vi "בדיקת מתח תפיסה של סליל פיקוד ללא עומס 4.vi"(8 "error":errorcluster, 11 "Path for Log":path) -> (0 "error out":errorcluster, 1 "מצב ממסר פתוח/סגור":bool, 2 "מתח סגירת הממסר":dbl format="%.4f", 3 "מתח מוצא מהספק":dbl format="%.4f", 5 "resultUserPrompt":bool)   [LabVIEW 2014]
uses:
  <vilib>/DAQmx/create/channels.llb/DAQmx Create Channel (DO-Digital Output).vi
  <vilib>/DAQmx/write.llb/DAQmx Write (Digital Bool 1Line 1Point).vi
panel:
  out "progress":dbl(slide) scale=0.0..36.0
  out "error IO DMM":errorcluster
  in  "Stop Button":bool
  # "Right-Click to\nexplain error"
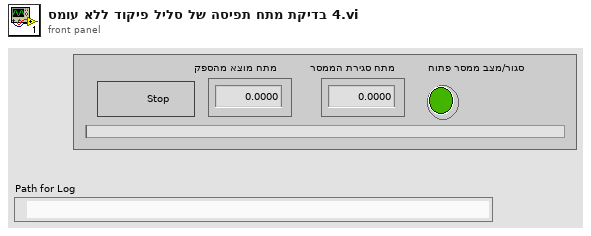
[diagram p1: front panel]
types:
  T1 = enum32{"Invalid", "Standard", "Closed", "Hidden", "Minimized", "Maximized"}
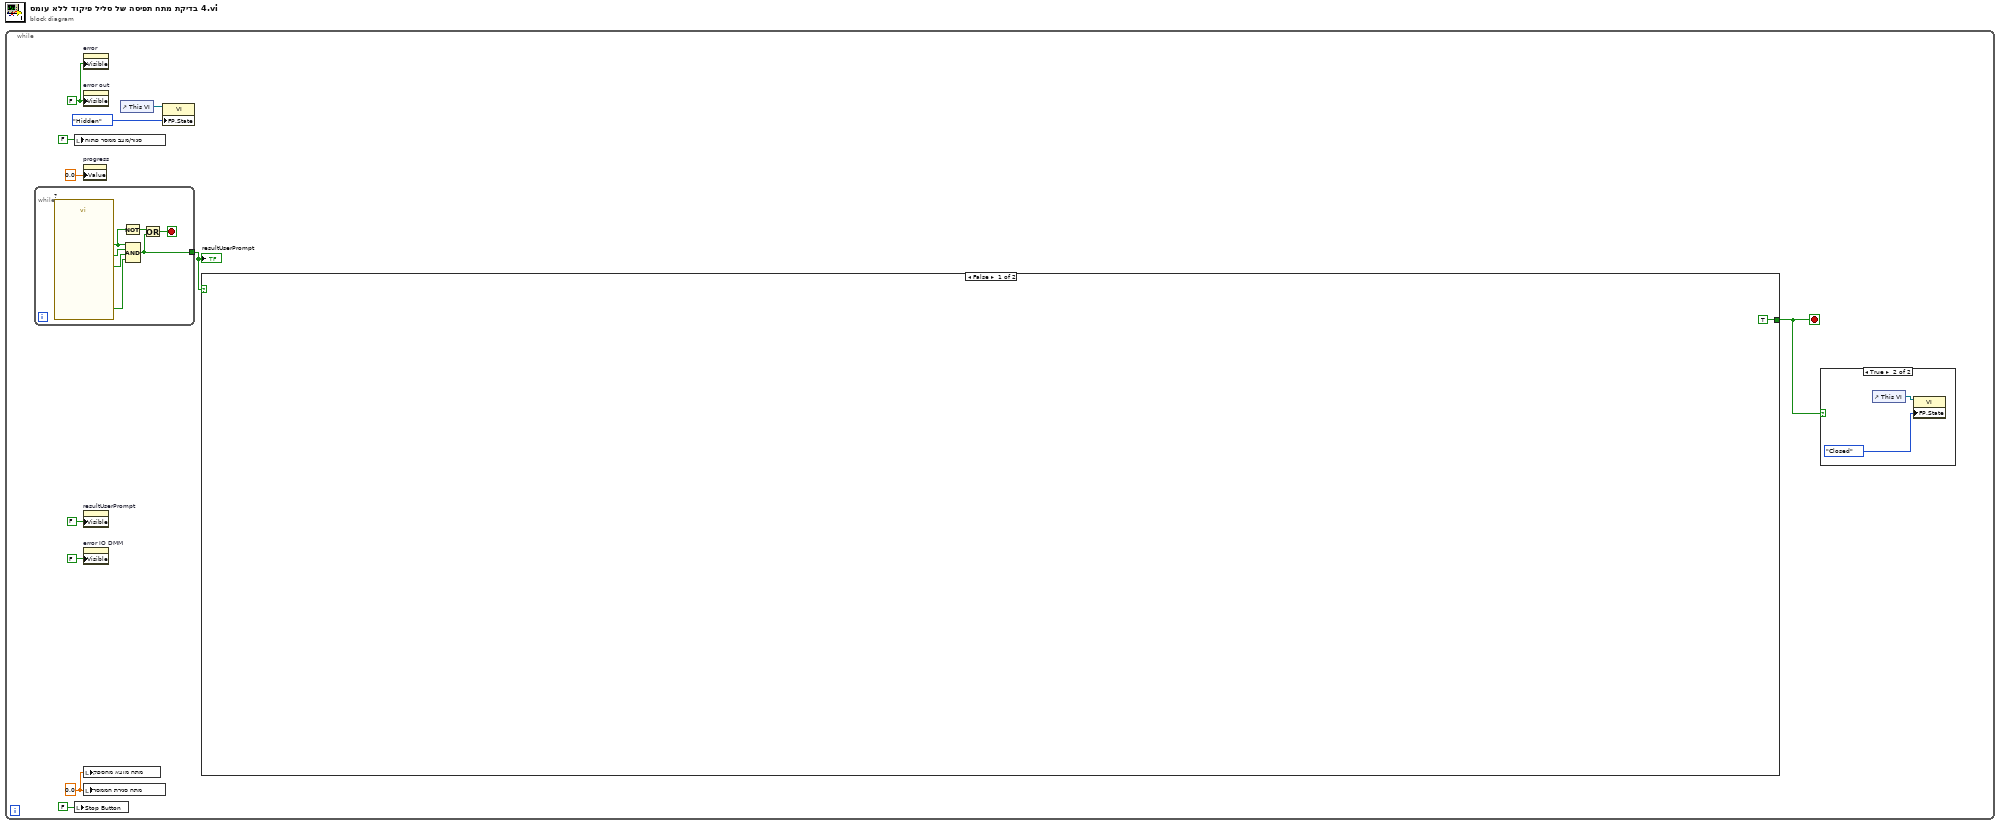
[diagram p0: block diagram]
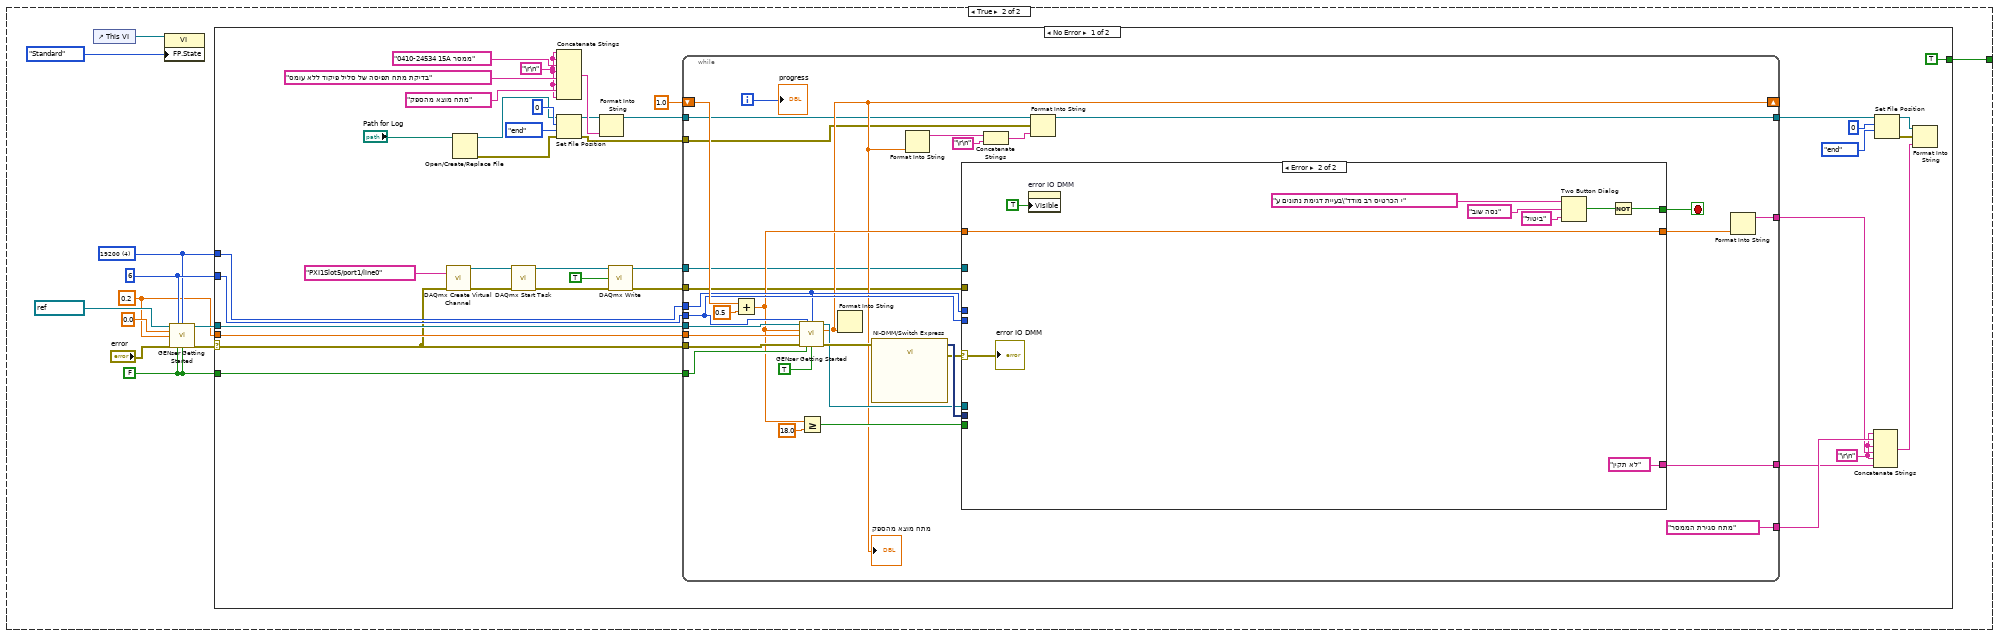
[diagram p3: hidden frame]
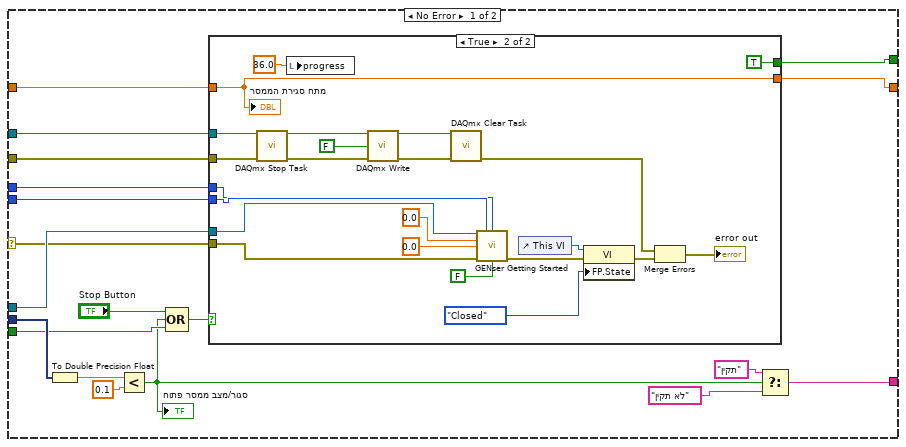
[diagram p4: hidden frame]
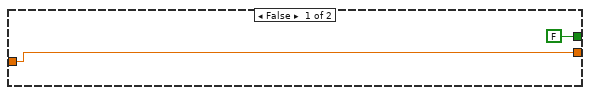
[diagram p5: hidden frame]
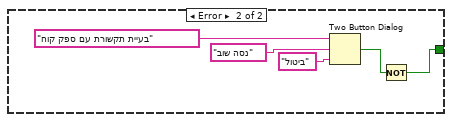
[diagram p6: hidden frame]
diagram:
  n1 = while {
    stop <- w1 stop-if-true
    w3 = FALSE ("Visible")
    w6 = 0.0 ("signals out")
    n2 = while {
      tunnel: [w12] -> w11
      stop <- w15 stop-if-true
      n3 = call "?"() -> ("הדקי הרב מודד"=w16:bool, "(מגע שלילי (מעטפת"=w17:bool, "A מגע חיובי"=w18:bool, "OK"=w13:bool)  [unwired: 15 in, 1 out]
      n4 = Not(x=w13) -> (.not. x?=w14:bool)
      n5 = Compound Arithmetic op=AND(w13, w18, w17, w16) -> (w12:bool)
      n6 = Or(x=w14, y=w12) -> (x .or. y?=w15:bool)
    }
    "resultUserPrompt" <- w11
    n7 = local write "מצב ממסר פתוח/סגור"(FALSE ("מגע סגור")) -> ()
    n8 = local write "Stop Button"(FALSE ("Reset (T)")) -> ()
    n9 = property on="error" class="Clust (strict)"("Visible"=w3) -> ()  [unwired: 2 in, 2 out]
    n10 = property on="error out" class="Clust (strict)"("Visible"=w3) -> ()  [unwired: 2 in, 2 out]
    n11 = property on="progress" class="Slide (strict)"("Value"=0.0 ("progress")) -> ()  [unwired: 2 in, 2 out]
    n12 = property on="resultUserPrompt" class="Bool (strict)"("Visible"=FALSE) -> ()  [unwired: 2 in, 2 out]
    n13 = property on="error IO DMM" class="Clust (strict)"("Visible"=FALSE) -> ()  [unwired: 2 in, 2 out]
    n14 = local write "מתח מוצא מהספק"(w6) -> ()
    n15 = local write "מתח סגירת הממסר"(w6) -> ()
    n16 = control-ref of="This VI"() -> (w5:refnum<vi>)
    n17 = property class="VI"(reference=w5, "FP.State"=T1."Hidden" ("Front Panel Window:State")) -> ()  [unwired: 1 in, 2 out]
    n18 = case shown="False" w11 {
      tunnel: [TRUE ("T button?") w27] -> w1
      frame False {
      }
      frame True {
        w26 = FALSE ("Output On (T)")
        w31 = u16 4 items=["1200", "2400", "4800", "9600", "19200"] ("BAUD")
        w32 = i16 6 ("GEN Addr")
        w28 = 0.2 ("Current Limit")
        n19 = control-ref of="This VI"() -> (w24:refnum<vi>)
        n20 = property class="VI"(reference=w24, "FP.State"=T1."Standard" ("Front Panel Window:State")) -> ()  [unwired: 1 in, 2 out]
        n21 = call "GENser Getting Started.vi"("VISA"=refnum<visa-resource-name> "COM6", "GEN Addr"=w32, "BAUD"=w31, "Voltage Limit"=0.0, "Current Limit"=w28, "error"="error", "Reset (T)"=w26, "Output On (T)"=w26) -> ("VISA out"=w33:refnum<visa-resource-name>, "error out"=w23:errorcluster)  [unwired: 4 in, 2 out]
        n22 = case shown="No Error" w23 {
          selector: w23 -> [w34 _]
          tunnel: w33 -> [w72 _]
          tunnel: w32 -> [w71 _]
          tunnel: w31 -> [w70 _]
          tunnel: w26 -> [w69 _]
          tunnel: w28 -> [w68 _]
          tunnel: [TRUE w157] -> w27
          frame No Error {
            w43 = "\r\n"
            w62 = "\r\n"
            n23 = call-poly <vilib>:"DAQmx Create Virtual Channel.vi"("lines"=tag "PXI1Slot5/port1/line0", "error in"=w34) -> ("task out"=w41:refnum<k21>, "error out"=w42:errorcluster)  [unwired: 12 in]
            n24 = Open/Create/Replace File(file path (use dialog)="Path for Log") -> (refnum out=w53:refnum<file>, error out=w52:errorcluster)  [unwired: 5 in, 1 out]
            n25 = call <vilib>:"DAQmx Start Task.vi"("task/channels in"=w41, "error in"=w42) -> ("task out"=w38:refnum<k21>, "error out"=w37:errorcluster)  [unwired: 12 in]
            n26 = Concatenate Strings(w43, w43, "0410-24534 15A ממסר", w43, "בדיקת מתח תפיסה של סליל פיקוד ללא עומס", w43, "מתח מוצא מהספק", w43) -> (w49:string)
            n27 = Set File Position(offset (in bytes) (0)=i64 0, refnum=w53, from (0:start)=enum16{"start", "end", "current"}."end", error in=w52) -> (refnum out=w45:refnum<file>, error out=w50:errorcluster)
            n28 = Format Into String(initial string=w45, w49) -> (resulting string=w44:refnum<file>)  [unwired: 2 in, 1 out]
            n29 = call-poly <vilib>:"DAQmx Write.vi"("task/channels in"=w38, "data"=TRUE, "error in"=w37) -> ("task out"=w36:refnum<k21>, "error out"=w35:errorcluster)  [unwired: 10 in, 1 out]
            n30 = while {
              tunnel: w72 -> [w92]
              tunnel: w34 -> [w103]
              tunnel: w71 -> [w94]
              tunnel: w70 -> [w93]
              tunnel: w69 -> [w102]
              tunnel: w68 -> [w100]
              shift-right: [w84] -> _
              shift-left: 1.0 ("y") -> [w98]
              tunnel: ["מתח סגירת הממסר"] -> w65
              tunnel: [w82] -> w64
              tunnel: [w81] -> w63
              tunnel: [w78] -> w61
              tunnel: w44 -> [w77]
              tunnel: w50 -> [w76]
              tunnel: w36 -> [w74]
              tunnel: w35 -> [w73]
              i -> [w85]
              stop <- w95 stop-if-true
              n31 = Add(x=w98, y=0.5) -> (x+y=w86:dbl)
              n32 = call "GENser Getting Started.vi"("VISA"=w92, "GEN Addr"=w94, "BAUD"=w93, "Voltage Limit"=w86, "Current Limit"=w100, "error"=w103, "Reset (T)"=w102, "Output On (T)"=TRUE) -> ("VISA out"=w91:refnum<visa-resource-name>, "Output Voltage"=w84:dbl, "error out"=w97:errorcluster)  [unwired: 4 in, 1 out]
              "מתח מוצא מהספק" <- w84
              n33 = Greater Or Equal?(x=w86, y=18.0) -> (x >= y?=w89:bool)
              n34 = Format Into String(w84) -> ()  [unwired: 3 in, 2 out]
              n35 = call "NI-DMM/Switch Express"("error in"=w97) -> ("signals out"=w96:dynamicdata, "error out"=w88:errorcluster)  [unwired: 16 in, 1 out]
              n36 = Format Into String(w84) -> (resulting string=w79:string)  [unwired: 3 in, 1 out]
              n37 = case shown="Error" w88 {
                selector: w88 -> [w114 w156]
                tunnel: w96 -> [w122 _]
                tunnel: [w111 w148] -> w95
                tunnel: w94 -> [w119 _]
                tunnel: w93 -> [w118 _]
                tunnel: w91 -> [w117 _]
                tunnel: w89 -> [w116 _]
                tunnel: w86 -> [w115 w151]
                tunnel: [w110 w151] -> w87
                tunnel: [w107 "לא תקין"] -> w81
                tunnel: w74 -> [w105 _]
                tunnel: w73 -> [w104 _]
                frame No Error {
                  n38 = To Double Precision Float(number=w122) -> (double precision float=w113:dbl)
                  n39 = Less?(x=w113, y=0.1) -> (x < y?=w106:bool)
                  "מצב ממסר פתוח/סגור" <- w106
                  n40 = Compound Arithmetic op=OR("Stop Button", w106, w116) -> (w121:bool)
                  n41 = case shown="True" w121 {
                    tunnel: [FALSE TRUE] -> w111
                    tunnel: w119 -> [_ w147]
                    tunnel: w118 -> [_ w146]
                    tunnel: w117 -> [_ w145]
                    tunnel: w114 -> [_ w142]
                    tunnel: w115 -> [w123 w137]
                    tunnel: [w123 w137] -> w110
                    tunnel: w105 -> [_ w127]
                    tunnel: w104 -> [_ w126]
                    frame False {
                    }
                    frame True {
                      n42 = call <vilib>:"DAQmx Stop Task.vi"("task/channels in"=w127, "error in"=w126) -> ("task out"=w135:refnum<k21>, "error out"=w133:errorcluster)  [unwired: 12 in]
                      n43 = local write "progress"(36.0 ("progress")) -> ()
                      n44 = call-poly <vilib>:"DAQmx Write.vi"("task/channels in"=w135, "data"=FALSE, "error in"=w133) -> ("task out"=w132:refnum<k21>, "error out"=w131:errorcluster)  [unwired: 10 in, 1 out]
                      n45 = call <vilib>:"DAQmx Clear Task.vi"("task in"=w132, "error in"=w131) -> ("error out"=w128:errorcluster)  [unwired: 13 in]
                      n46 = call "GENser Getting Started.vi"("VISA"=w145, "GEN Addr"=w147, "BAUD"=w146, "Voltage Limit"=0.0, "Current Limit"=0.0, "error"=w142, "Output On (T)"=FALSE) -> ("error out"=w125:errorcluster)  [unwired: 5 in, 3 out]
                      n47 = control-ref of="This VI"() -> (w139:refnum<vi>)
                      n48 = property class="VI"(reference=w139, error in=w125, "FP.State"=T1."Closed" ("Front Panel Window:State")) -> (error out=w129:errorcluster)  [unwired: 1 out]
                      n49 = Merge Errors(w128, w129) -> (→"error out":errorcluster)
                      "מתח סגירת הממסר" <- w137
                    }
                  }
                  n50 = Select(t="תקין", s=w106, f="לא תקין") -> (s? t:f=w107:string)
                }
                frame Error {
                  n51 = property on="error IO DMM" class="Clust (strict)"("Visible"=TRUE) -> ()  [unwired: 2 in, 2 out]
                  n52 = Two Button Dialog(message="בעיית דגימת נתונים ע\"י הכרטיס רב מודד", 1:"ביטול" ("F button name (\"Cancel\")"), 2:"נסה שוב" ("T button name (\"OK\")")) -> (T button?=w149:bool)
                  n53 = Not(x=w149) -> (.not. x?=w148:bool)
                  "error IO DMM" <- w156
                }
              }
              n54 = Concatenate Strings(w79, "\r\n") -> (w75:string)
              n55 = Format Into String(initial string=w77, error in=w76, w75) -> (resulting string=w78:refnum<file>)  [unwired: 1 in, 1 out]
              n56 = Format Into String(w87) -> (resulting string=w82:string)  [unwired: 3 in, 1 out]
              "progress" <- w85
            }
            n57 = Concatenate Strings(w62, w65, w62, w64, w62, w63) -> (w56:string)
            n58 = Set File Position(offset (in bytes) (0)=i64 0, refnum=w61, from (0:start)=enum16{"start", "end", "current"}."end") -> (refnum out=w58:refnum<file>, error out=w57:errorcluster)  [unwired: 1 in]
            n59 = Format Into String(initial string=w58, error in=w57, w56) -> ()  [unwired: 1 in, 2 out]
          }
          frame Error {
            n60 = Two Button Dialog(message="בעיית תקשורת עם ספק קוח", 1:"ביטול" ("F button name (\"Cancel\")"), 2:"נסה שוב" ("T button name (\"OK\")")) -> (T button?=w158:bool)
            n61 = Not(x=w158) -> (.not. x?=w157:bool)
          }
        }
      }
    }
    n62 = case shown="True" w1 {
      frame False {
      }
      frame True {
        n63 = control-ref of="This VI"() -> (w19:refnum<vi>)
        n64 = property class="VI"(reference=w19, "FP.State"=T1."Closed" ("Front Panel Window:State")) -> ()  [unwired: 1 in, 2 out]
      }
    }
  }
